vi "read_COM_Port.vi"() -> ()   [LabVIEW 2020]
uses:
  <vilib>/Instr/_visa.llb/VISA Configure Serial Port (Instr).vi
  gVar_ECa1.vi
  gVar_ECa2.vi
  gVar_ECa3.vi
  gVar_ECa4.vi
panel:
  out "Array 2":dbl[](array[numeric])
  out "Array":dbl[](array[numeric])
  out "Samples per drop":dbl format="%#_4g"
  out "total counts":i32
  out "dropped samples":i32
  out "Loop Time (ms)":u32
  out "Waveform Chart 2":dbl(graph)
  out "ECa1 (generated)":dbl
  out "TSM-ECa":dbl
  out "Waveform Chart":dbl(graph)
  in  "ECa Chn":u8 max=3 step=1
  out "Bytes at COM":u32
  out "read buffer":string
  in  "stop":bool
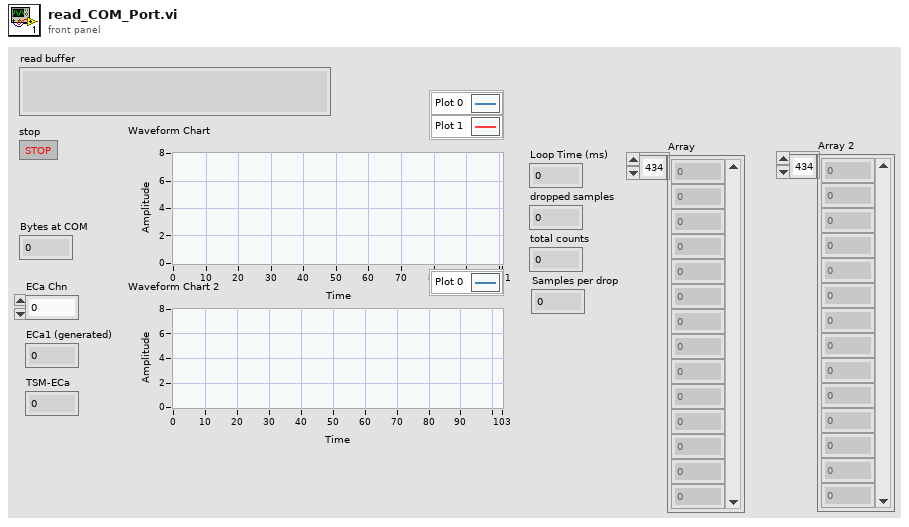
[diagram p1: front panel]
types:
  T1 = typedef "SensorData_TypDef.ctl" = cluster{"ECa":dbl[], "iP":dbl[], "IMU":dbl[], "iH":dbl[]}
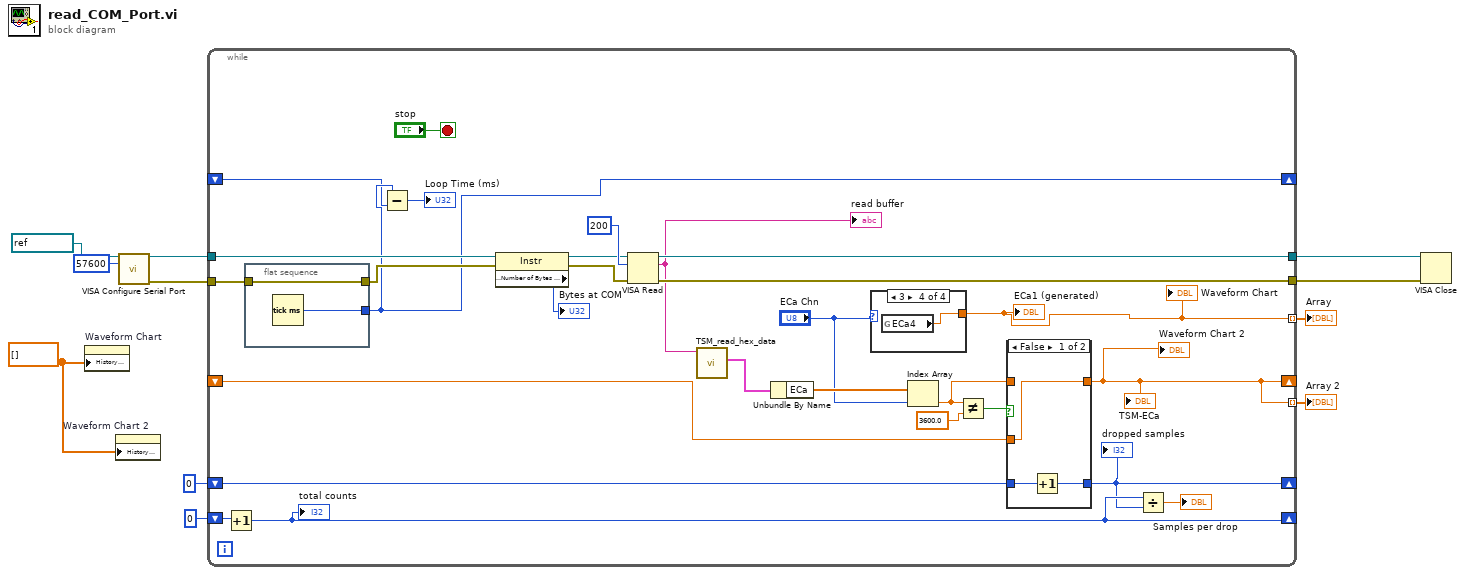
[diagram p0: block diagram]
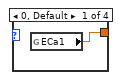
[diagram p2: hidden frame]
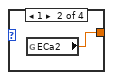
[diagram p3: hidden frame]
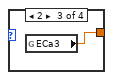
[diagram p4: hidden frame]
diagram:
  w6 = dbl[] [] ("History Data")
  n1 = property on="Waveform Chart" class="WFChart (strict)"("History Data"=w6) -> ()  [unwired: 2 in, 2 out]
  n2 = property on="Waveform Chart 2" class="WFChart (strict)"("History Data"=w6) -> ()  [unwired: 2 in, 2 out]
  n3 = call-poly "VISA Configure Serial Port"("VISA resource name"=refnum<visa-resource-name> "COM1", "baud rate (9600)"=u32 57600) -> ("VISA resource name out"=w11:refnum<visa-resource-name>, "error out"=w10:errorcluster)  [unwired: 12 in]
  n4 = while {
    tunnel: w11 -> [w35]
    tunnel: w10 -> [w25]
    tunnel: [w39] -> w7
    tunnel: [w38] -> w8
    shift-right: [w13] -> _
    shift-left: _ -> [w26]
    shift-right: [w22] -> _
    shift-left: _ -> [w21]
    shift-right: [w17] -> _
    shift-left: 0 -> [w20]
    shift-right: [w18] -> _
    shift-left: 0 -> [w19]
    tunnel: [w14] -> w2 mode=indexing
    tunnel: [w13] -> w1 mode=indexing
    stop <- "stop" stop-if-true
    n5 = Increment(x=w19) -> (x+1=w18:i32)
    "total counts" <- w18
    n6 = flat-sequence {
      tunnel: w25 -> [w45]
      tunnel: [w45] -> w24
      tunnel: [w44] -> w22
      frame #0 {
        n7 = Tick Count (ms)() -> (millisecond timer value=w44:u32)
      }
    }
    n8 = Subtract(x=w22, y=w21) -> (x-y=→"Loop Time (ms)":u32)
    n9 = property class="Instr"(reference=w35, error in=w24) -> (reference out=w34:refnum<visa-resource-name>, error out=w33:errorcluster, "Serial Settings:Number of Bytes at Serial Port"=→"Bytes at COM":u32)
    n10 = VISA Read(VISA resource name=w34, byte count=200, error in (no error)=w33) -> (VISA resource name out=w39:refnum<visa-resource-name>, read buffer=w31:string, error out=w38:errorcluster)  [unwired: 1 out]
    "read buffer" <- w31
    n11 = call "TSM_read_hex_data.vi"("read buffer in"=w31) -> ("SensorData"=w12:T1)  [unwired: 7 in, 3 out]
    n12 = Unbundle By Name(w12) -> ("ECa"=w30:dbl[])
    n13 = case shown="3" "ECa Chn" {
      tunnel: [w40 w41 w42 w43] -> w14
      frame 0, Default {
        n14 = global read "gVar_ECa1.vi" "ECa1"() -> (w40:dbl)
      }
      frame 1 {
        n15 = global read "gVar_ECa2.vi" "ECa2"() -> (w41:dbl)
      }
      frame 2 {
        n16 = global read "gVar_ECa3.vi" "ECa3"() -> (w42:dbl)
      }
      frame 3 {
        n17 = global read "gVar_ECa4.vi" "ECa4"() -> (w43:dbl)
      }
    }
    "Waveform Chart" <- w14
    "ECa1 (generated)" <- w14
    n18 = Index Array(array=w30, index="ECa Chn") -> (element=w27:dbl)
    n19 = Not Equal?(x=w27, y=3600.0) -> (x != y?=w28:bool)
    n20 = case shown="False" w28 {
      tunnel: [w48 w50] -> w13
      tunnel: w27 -> [_ w50]
      tunnel: w26 -> [w48 _]
      tunnel: [w47 w49] -> w17
      tunnel: w20 -> [w46 w49]
      frame False {
        n21 = Increment(x=w46) -> (x+1=w47:i32)
      }
      frame True {
      }
    }
    "TSM-ECa" <- w13
    "Waveform Chart 2" <- w13
    "dropped samples" <- w17
    n22 = Divide(x=w18, y=w17) -> (x/y=→"Samples per drop":dbl)
  }
  "Array" <- w2
  "Array 2" <- w1
  n23 = VISA Close(VISA resource name=w7, error in (no error)=w8) -> ()  [unwired: 1 out]
